vi "_05_06_05_PM.vi"() -> ()   [LabVIEW 2020]
panel:
  in  "?":cluster{}
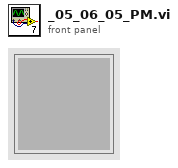
[diagram p1: front panel]
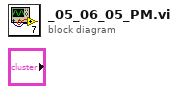
[diagram p0: block diagram]
diagram:
